vi "Estrai funz correttrice.vi"(9 "nome canale":string, 10 "Assoc_input_sensori":string[][](array[string]), 11 "canale--sensore":string[][](array[string])) -> (0 "conv. con range offset":T2, 1 "INTERPOLAZIONE SETTINGS":T3, 2 "USA FUNZ CORR":bool, 3 "FUNZ CORR PRESENTE":bool, 4 "um":i32)   [LabVIEW 2019]
panel:
  in  "Unità di Misura":T1
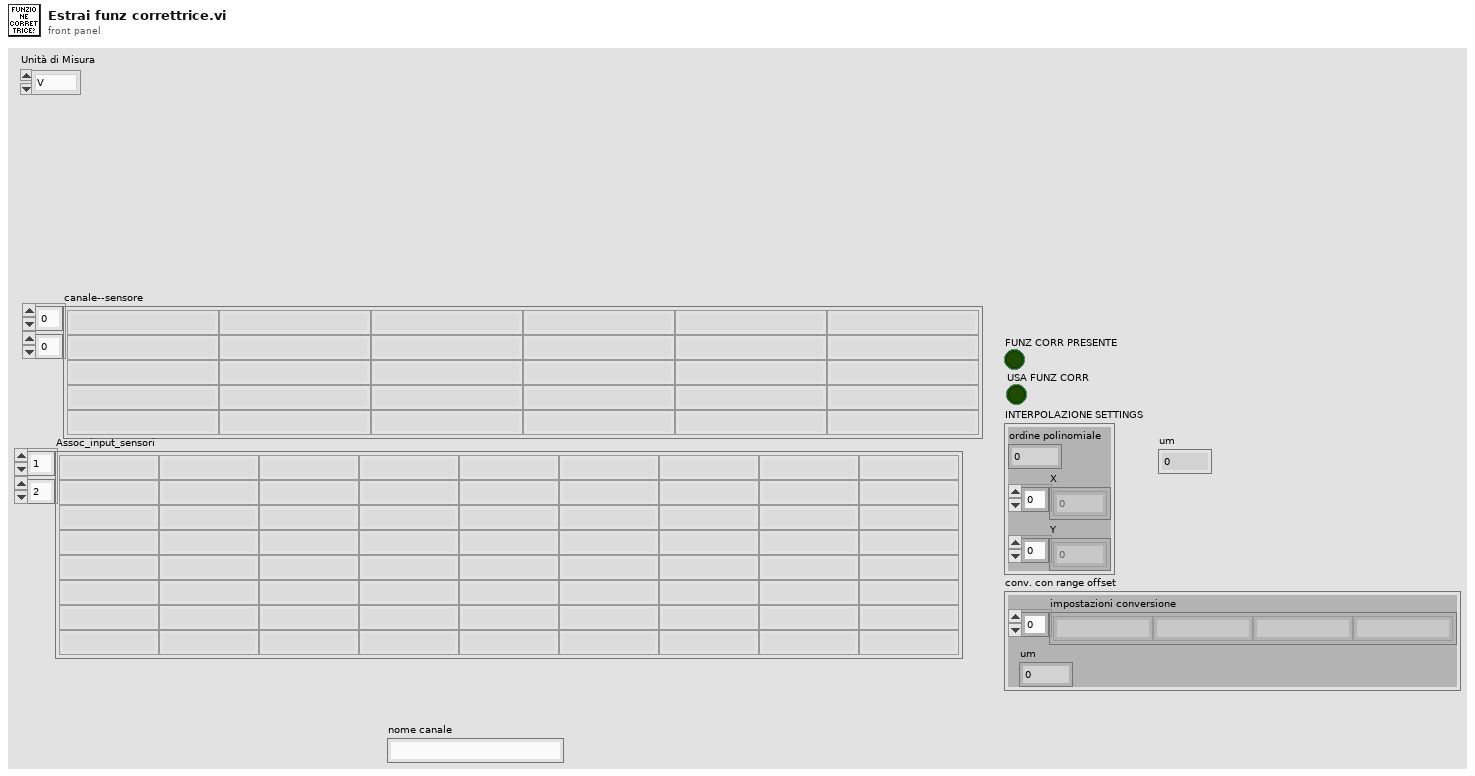
[diagram p1: front panel]
types:
  T1 = typedef "UnitàMisura.ctl" = enum16{"V", "mA", "Bar", "RPM", "m3/s", "m3/min", "m3/h", "l/s", "l/min", "in3/min", "ft3/min", "gpm", "igpm", "igph", "%", "°C", "m", "Nm", "A"}
  T2 = cluster{"impostazioni conversione":string[], "um":i32}
  T3 = cluster{"ordine polinomiale":i32, "X":dbl[], "Y":dbl[]}
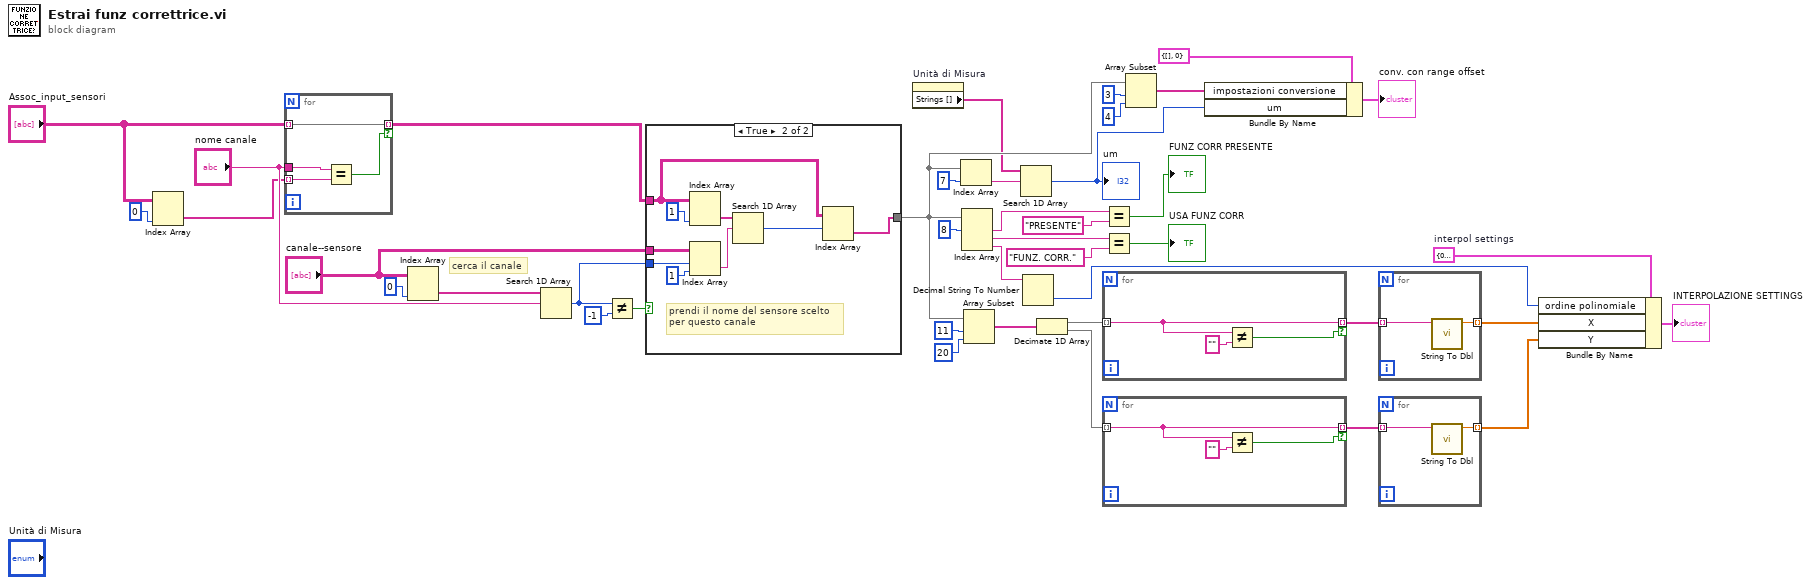
[diagram p0: block diagram]
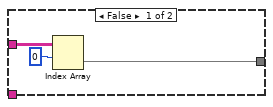
[diagram p2: hidden frame]
diagram:
  w22 = T3 {"ordine polinomiale"=0, "X"=[], "Y"=[]}  # interpol settings
  # "cerca il canale"
  n1 = Index Array(array="Assoc_input_sensori", index (col)=0 ("disabled index (col)")) -> (element=w32:string[])  [unwired: 1 in]
  n2 = for {
    tunnel: w32 -> [w45] mode=indexing
    tunnel: [w42] -> w38 mode=indexing if=w43
    tunnel: "nome canale" -> [w44]
    tunnel: "Assoc_input_sensori" -> [w42] mode=indexing
    n3 = Equal?(x=w44, y=w45) -> (x = y?=w43:bool)
  }
  n4 = Index Array(array="canale--sensore", index (col)=0 ("disabled index (col)")) -> (element=w35:string[])  [unwired: 1 in]
  n5 = Search 1D Array(1D array=w35, element="nome canale") -> (index of element=w39:i32)  [unwired: 1 in]
  n6 = Not Equal?(x=w39, y=-1) -> (x != y?=w41:bool)
  n7 = case shown="True" w41 {
    tunnel: "canale--sensore" -> [_ w56]
    tunnel: w38 -> [w48 w51]
    tunnel: w39 -> [_ w50]
    tunnel: [w46 w49] -> w11
    frame False {
      n8 = Index Array(array=w48, index (row)=0) -> (element=w46:string[])  [unwired: 1 in]
    }
    frame True {
      # "prendi il nome del sensore scelto\nper questo canale"
      n9 = Index Array(array=w51, index (col)=1 ("disabled index (col)")) -> (element=w54:string[])  [unwired: 1 in]
      n10 = Index Array(array=w56, index (row)=w50, index (col)=1 ("disabled index (col)")) -> (element=w53:string)
      n11 = Search 1D Array(1D array=w54, element=w53) -> (index of element=w52:i32)  [unwired: 1 in]
      n12 = Index Array(array=w51, index (row)=w52) -> (element=w49:string[])  [unwired: 1 in]
    }
  }
  n13 = property on="Unità di Misura" class="Enum (strict)"() -> ("Strings []"=w8:string[])  [unwired: 2 in, 2 out]
  n14 = Index Array(array=w11, index=7) -> (element=w7:string)
  n15 = Index Array(array=w11, index #1=8 ("index")) -> (element #1=w29:string, element #2=w26:string, element #3=w23:string)  [unwired: 2 in]
  n16 = Array Subset(array=w11, index=11, length=20) -> (w19:string[])
  n17 = Search 1D Array(1D array=w8, element=w7) -> (index of element=w6:i32)  [unwired: 1 in]
  "um" <- w6
  n18 = Decimal String To Number(string=w23) -> (number=w1:i32)  [unwired: 2 in, 1 out]
  n19 = Decimate 1D Array(w19) -> (w5:string[], w3:string[])
  n20 = for {
    tunnel: w5 -> [w60] mode=indexing
    tunnel: [w60] -> w4 mode=indexing if=w59
    n21 = Not Equal?(x=w60, y="") -> (x != y?=w59:bool)
  }
  n22 = for {
    tunnel: w3 -> [w63] mode=indexing
    tunnel: [w63] -> w2 mode=indexing if=w62
    n23 = Not Equal?(x=w63, y="") -> (x != y?=w62:bool)
  }
  n24 = Equal?(x=w29, y="PRESENTE") -> (x = y?=→"FUNZ CORR PRESENTE":bool)
  n25 = Equal?(x=w26, y="FUNZ. CORR.") -> (x = y?=→"USA FUNZ CORR":bool)
  n26 = Array Subset(array=w11, index=3, length=4) -> (w12:string[])
  n27 = Bundle By Name(cluster=T2 {"impostazioni conversione"=[], "um"=0}, "impostazioni conversione"=w12, "um"=w6) -> (→"conv. con range offset":T2)
  n28 = for {
    tunnel: w4 -> [w65] mode=indexing
    tunnel: [w64] -> w18 mode=indexing
    n29 = call "String To Dbl.vi"("String"=w65) -> ("Numeric"=w64:dbl)  [unwired: 10 in]
  }
  n30 = for {
    tunnel: w2 -> [w67] mode=indexing
    tunnel: [w66] -> w17 mode=indexing
    n31 = call "String To Dbl.vi"("String"=w67) -> ("Numeric"=w66:dbl)  [unwired: 10 in]
  }
  n32 = Bundle By Name(cluster=w22, "ordine polinomiale"=w1, "X"=w18, "Y"=w17) -> (→"INTERPOLAZIONE SETTINGS":T3)
